vi "Insert.vi"(8 "error in (no error)":errorcluster, 9 "String":string, 10 "Index":i32, 11 "StringList in":refnum<class "StringList.lvclass">) -> (0 "error out":errorcluster, 3 "StringList out":refnum<class "StringList.lvclass">)   [LabVIEW 2013, in "LapDog.Collections.v_.Lists.lvlib" / "StringList.lvclass"]
uses:
  StringList.lvclass
  ObjectList/ObjectList.lvclass
  LapDog.Collections.Common/String/String.lvclass
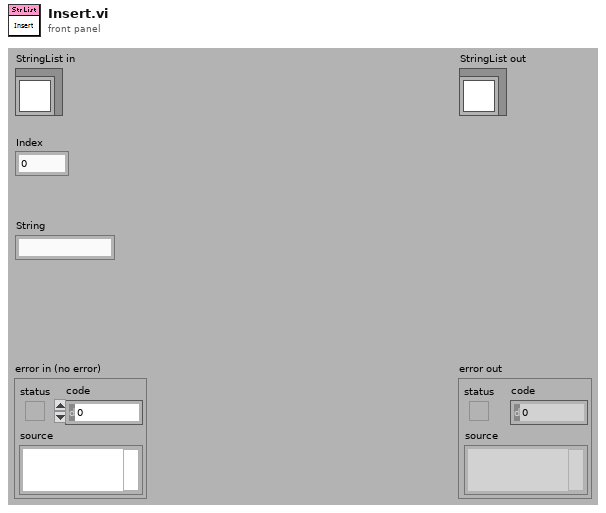
[diagram p1: front panel]
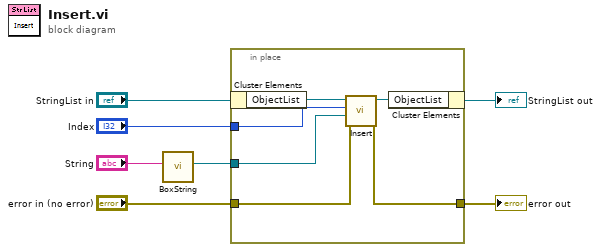
[diagram p0: block diagram]
diagram:
  n1 = call "BoxString.vi"("String"="String") -> ("String out"=w3:refnum<class "String.lvclass">)  [unwired: 10 in]
  n2 = in-place {
    in-place-border: "Index" -> [w11]
    in-place-border: w3 -> [w10]
    in-place-border: "error in (no error)" -> [w9]
    in-place-border: [w8] -> w1
    n3 = in-place-cluster #1("StringList in") -> ("ObjectList"=w13:refnum<class "ObjectList.lvclass">)
    n4 = call-dynamic "Insert.vi"("error in (no error)"=w9, "Item"=w10, "Index"=w11, "List in"=w13) -> ("error out"=w8:errorcluster, "List out"=w12:refnum<class "ObjectList.lvclass">)  [unwired: 6 in]
    n5 = in-place-cluster #1("ObjectList"=w12) -> (→"StringList out":refnum<class "StringList.lvclass">)
  }
  "error out" <- w1
